vi "Acquisition Query.vi"(8 "error in":errorcluster, 11 "Instrument Handle In":i32) -> (0 "error out":errorcluster, 1 "Acquire Count":i32, 2 "Acquire Type":i32, 3 "Instrument Handle Out":i32, 4 "Initiate Continuously":i32, 5 "Trigger Mode":i32)   [LabVIEW 8.6, in "ZTScopeM.lvlib"]
doc: "Query the acquisition settings of the oscilloscope."
uses:
  ZTScopeM.lvlib
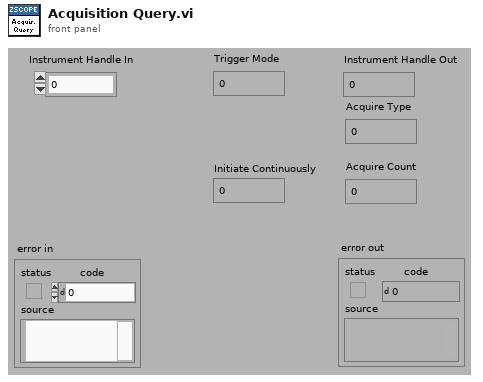
[diagram p1: front panel]
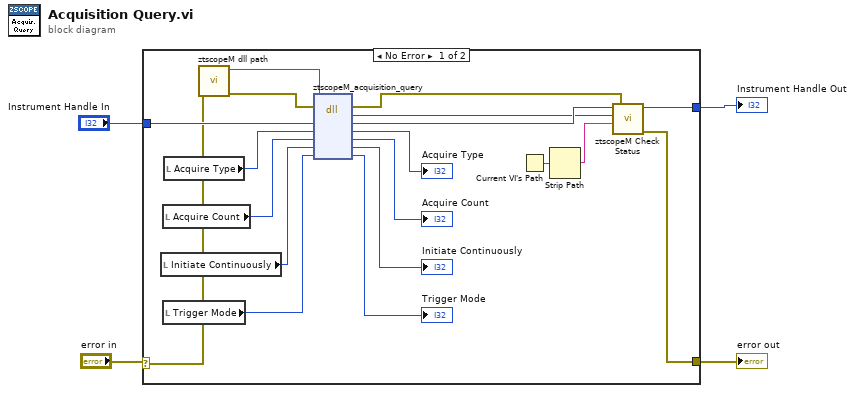
[diagram p0: block diagram]
diagram:
  n1 = case shown="No Error" "error in" {
    selector: "error in" -> [w8 w25]
    tunnel: [w10 w25] -> w1
    tunnel: "Instrument Handle In" -> [w23 w24]
    tunnel: [w9 w24] -> w3
    frame #0 {
      n2 = local read "Initiate Continuously"() -> (w18:i32)
      n3 = local read "Acquire Count"() -> (w20:i32)
      n4 = local read "Trigger Mode"() -> (w16:i32)
      n5 = local read "Acquire Type"() -> (w22:i32)
      n6 = call "ztscopeM dll path.vi"("error in (no error)"=w8) -> ("error out"=w6:errorcluster, "<instrument>.dll path"=w7:path)  [unwired: 9 in]
      n7 = dll-call lib="C:/Program Files (x86)/National Instruments/LabVIEW 2013/instr.lib/ztscopem/ztscopeM.dll" fn="ztscopeM_acquisition_query"(path in=w7, error in=w6, "instrumentHandle"=w23, "acquireType"=w22, "acquireCount"=w20, "initiateContinuously"=w18, "triggerMode"=w16) -> (error out=w5:errorcluster, w11:i32, "instrumentHandle"=w12:i32, "acquireType"=→"Acquire Type":i32, "acquireCount"=→"Acquire Count":i32, "initiateContinuously"=→"Initiate Continuously":i32, "triggerMode"=→"Trigger Mode":i32)  [unwired: 1 in, 1 out]
      n8 = Current VI's Path() -> (path=w14:path)
      n9 = Strip Path(path=w14) -> (name=w13:string)  [unwired: 1 out]
      n10 = call "ztscopeM Check Status.vi"("error in"=w5, "name of VI"=w13, "status (return code)"=w11, "instrument handle in"=w12) -> ("error out"=w10:errorcluster, "instrument handle out"=w9:i32)  [unwired: 2 in]
    }
    frame #1 {
    }
  }
  "Instrument Handle Out" <- w3
  "error out" <- w1
